vi "CheckZLUTDimensions.vi"(10 "ZLUT":sgl[][][](array[numeric]), 11 "MeasureConfig":T1={"Bead locations"=[{"X"=0, "Y"=0}], "ROI"=200, "Experiment base path"=path "", "Image output subdir"="images", "Output mode"=enum."None", "Traces output subdir"="traces", "QTrk Settings"={"Image width"=150, "Image height"=150, "Number of threads (CPU based)"=-1, "CUDA Device"=-2, "COM Background correction factor"=0.0, "ZLUT MinRadius"=8.0, "ZLUT Radial sample density"=5.0, "ZLUT Angular sample density"=2.0, "ZLUT ROI Coverage"=0.7, "QI Iterations"=1, "QI MinRadius"=2.0, "QI Radial sample density"=5.0, "QI Angular sample density"=2.0, "QI ROI Coverage"=0.7, "QI Angular Step \nIteration Factor"=0.8, "XCOR Profile Length"=1, "XCOR Profile Width"=128, "XCOR Iterations"=32, "Gaussian 2D Fit Iterations"=2, "Gaussian 2D Sigma (pixels)"=3.0, "Downsample"=0}, "Tracking Config"={"Number of steps"=0, "ZLUT stepsize (um)"=0.0, "Z correction factor"=0.0, "Start piezo Z (um)"=0.0, "Pixel size (nm)"=0.0, "2D Localization Type"=enum."Quadrant Interpolation", "Z Command (None)"=enum."Nothing", "Z Piezo scale"=FALSE}, "Experiment Name"="", "Program"={"Commands"=[], "Motor Axis accuracy conditions"={"Magnet Z"=0.0, "Magnet rotation"=0.0, "Camera"={"X"=0.0, "Y"=0.0}, "Piezo XY"={"X"=0.0, "Y"=0.0}, "Piezo Z"=0.0}, "Axis flags"={"Magnet Z"=FALSE, "Magnet rotation"=FALSE, "Camera"={"X"=FALSE, "Y"=FALSE}, "Piezo XY"={"X"=FALSE, "Y"=FALSE}, "Piezo Z"=FALSE}}, "ZLUT"=[], "Camera settings"={"Framerate (Hz)"=60, "Exposure time (us)"=5000, "Image size"={"Width"=1280, "Height"=1024}, "Number of buffers"=30}, "Experiment Script"="", "Max frames in memory"=2, "Save traces as binary"=FALSE, "Pixel Calibration Gain Image"="camera_calib_gain.bin", "Pixel Calibration Offset Image"="camera_calib_gain.bin", "Use pixel calibration images"=FALSE, "Internal camera settings"="", "Trace write interval"=100} {"QTrk Settings"."QI ROI Coverage" format="%_2g"; "QTrk Settings"."QI MinRadius" format="%.2f"; "QTrk Settings"."QI Angular sample density" format="%.3f"; "QTrk Settings"."QI Radial sample density" format="%.2f"; "QTrk Settings"."ZLUT Radial sample density" format="%.2f"; "QTrk Settings"."ZLUT MinRadius" format="%.2f"}) -> (2 "OK?":bool)   [LabVIEW 2011]
uses:
  Typedefs/MeasureConfigType.ctl
  Typedefs/MeasureConfigOutputMode.ctl
  qtrk/QTrkLVBinding/QTrkSettings.ctl
  Typedefs/TrackingConfigType.ctl
  qtrk/QTrkLVBinding/QTrkLocalizationType.ctl
  qtrk/QTrkLVBinding/QTrkZCommandType.ctl
  ExperimentProgram/ExperimentProgramType.ctl
  ExperimentProgram/ExProgCommandType.ctl
  ExperimentProgram/ExProgCommandEnumType.ctl
  Motors/MotorAxisEnum.ctl
  Motors/MotorPosType.ctl
  Typedefs/XYf.ctl
  Motors/MotorPosFlagsType.ctl
  Camera/GenericCameraConfigType.ctl
panel:
  # "(used for commands with string parameters)"
  # "-2: Use all devices\n-1: Use best device"
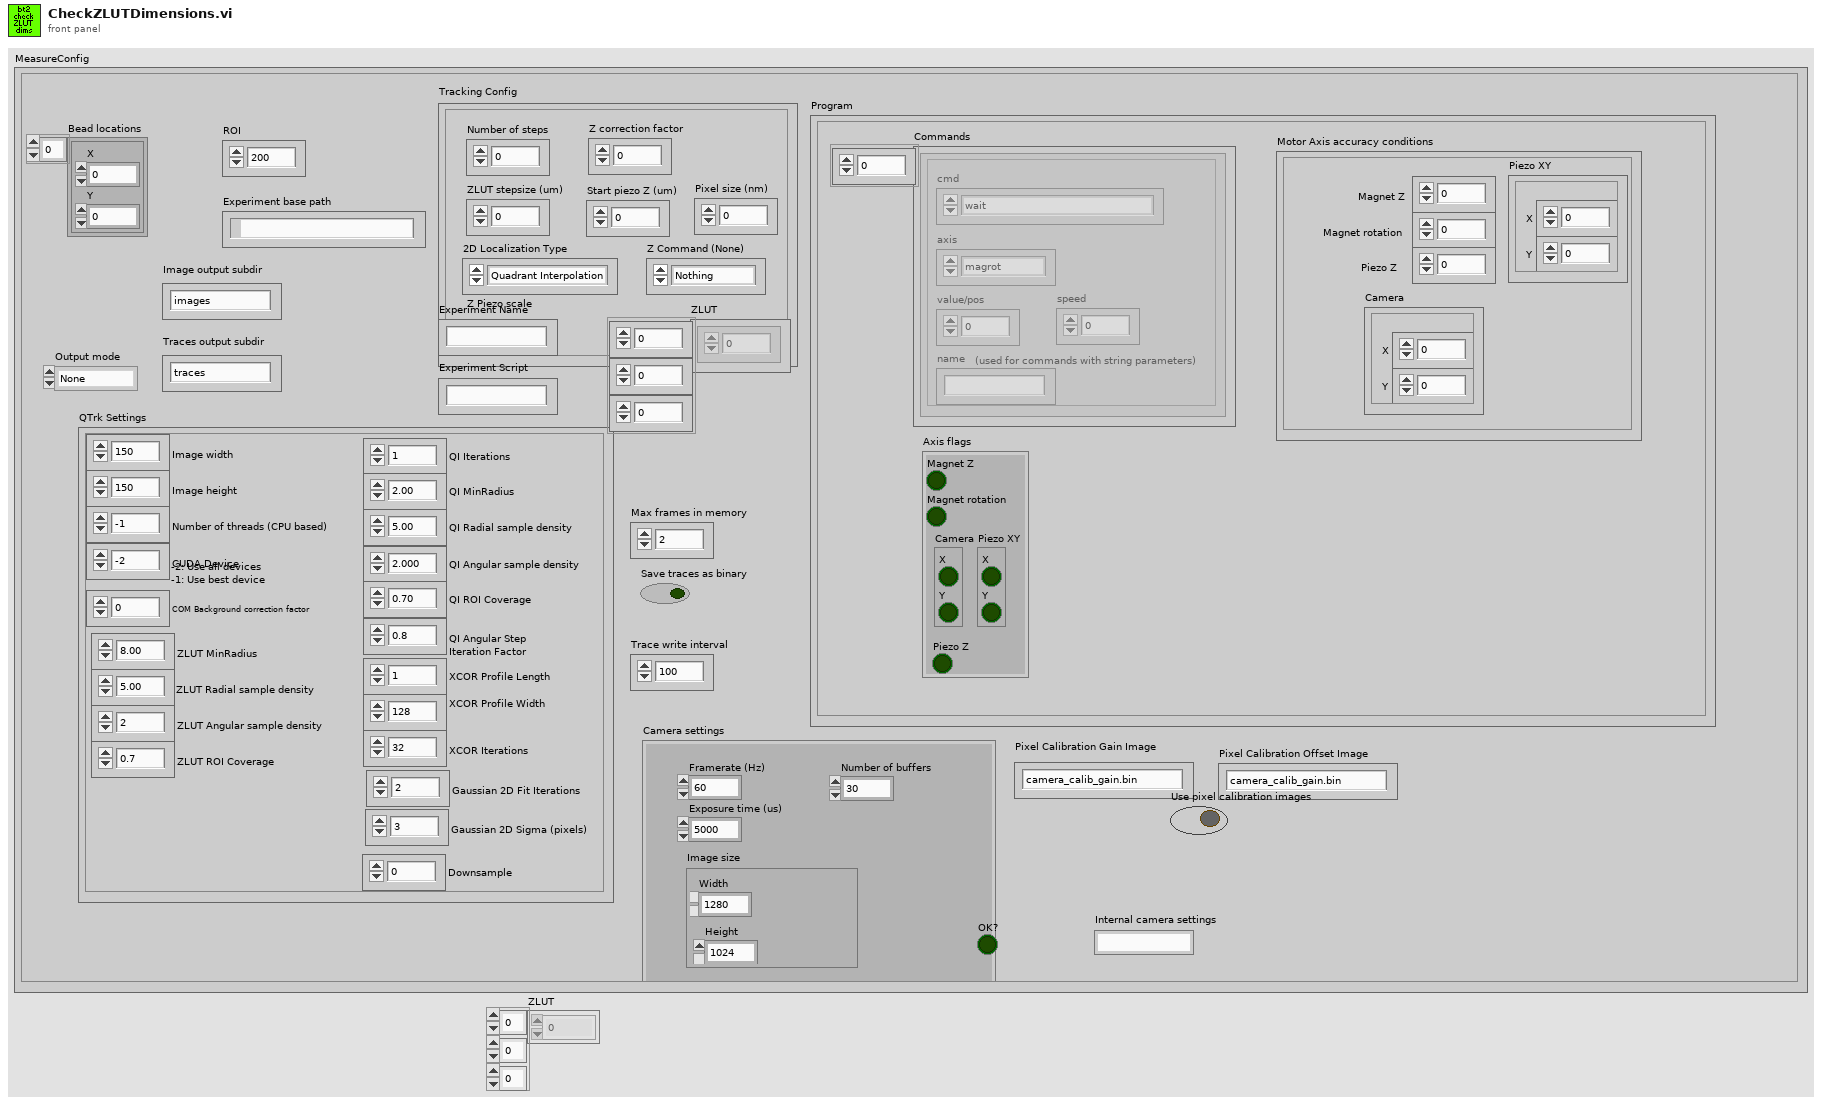
[diagram p1: front panel]
types:
  T1 = typedef "MeasureConfigType.ctl" = cluster{"Bead locations":cluster{"X":i32, "Y":i32}[], "ROI":i32, "Experiment base path":path, "Image output subdir":string, "Output mode":T2, "Traces output subdir":string, "QTrk Settings":T3, "Tracking Config":T4, "Experiment Name":string, "Program":T7, "ZLUT":sgl[][][], "Camera settings":T14, "Experiment Script":string, "Max frames in memory":i32, "Save traces as binary":bool, "Pixel Calibration Gain Image":string, "Pixel Calibration Offset Image":string, "Use pixel calibration images":bool, "Internal camera settings":string, "Trace write interval":i32}
  T2 = typedef "MeasureConfigOutputMode.ctl" = enum16{"None", "Track", "SaveImages"}
  T3 = typedef "QTrkSettings.ctl" = cluster{"Image width":i32, "Image height":i32, "Number of threads (CPU based)":i32, "CUDA Device":i32, "COM Background correction factor":sgl, "ZLUT MinRadius":sgl, "ZLUT Radial sample density":sgl, "ZLUT Angular sample density":sgl, "ZLUT ROI Coverage":sgl, "QI Iterations":i32, "QI MinRadius":sgl, "QI Radial sample density":sgl, "QI Angular sample density":sgl, "QI ROI Coverage":sgl, "QI Angular Step \nIteration Factor":sgl, "XCOR Profile Length":i32, "XCOR Profile Width":i32, "XCOR Iterations":i32, "Gaussian 2D Fit Iterations":i32, "Gaussian 2D Sigma (pixels)":sgl, "Downsample":i32}
  T4 = typedef "TrackingConfigType.ctl" = cluster{"Number of steps":i32, "ZLUT stepsize (um)":sgl, "Z correction factor":sgl, "Start piezo Z (um)":sgl, "Pixel size (nm)":sgl, "2D Localization Type":T5, "Z Command (None)":T6, "Z Piezo scale":bool}
  T5 = typedef "QTrkLocalizationType.ctl" = enum16{"Center-of-Mass", "1D Cross-Correlation", "Quadrant Interpolation", "Gaussian 2D MLE", "QI + ZLUTAlign", "ZLUTAlign", "QI + FourierLUT"}
  T6 = typedef "QTrkZCommandType.ctl" = enum16{"Nothing", "ComputeZ", "BuildRadialZLUT", "BuildImageZLUT", "RadialZLUT+ImageZLUT"}
  T7 = typedef "ExperimentProgramType.ctl" = cluster{"Commands":T8[], "Motor Axis accuracy conditions":T11, "Axis flags":T13}
  T8 = typedef "ExProgCommandType.ctl" = cluster{"cmd":T9, "axis":T10, "value/pos":dbl, "speed":dbl, "name":string}
  T9 = typedef "ExProgCommandEnumType.ctl" = enum16{"wait", "move", "acquire", "idle", "rmove", "when", "section", "stop"}
  T10 = typedef "MotorAxisEnum.ctl" = enum16{"no axis", "magrot", "magpos", "px", "py", "pz", "camx", "camy"}
  T11 = typedef "MotorPosType.ctl" = cluster{"Magnet Z":dbl, "Magnet rotation":dbl, "Camera":T12, "Piezo XY":T12, "Piezo Z":dbl}
  T12 = typedef "XYf.ctl" = cluster{"X":sgl, "Y":sgl}
  T13 = typedef "MotorPosFlagsType.ctl" = cluster{"Magnet Z":bool, "Magnet rotation":bool, "Camera":cluster{"X":bool, "Y":bool}, "Piezo XY":cluster{"X":bool, "Y":bool}, "Piezo Z":bool}
  T14 = typedef "GenericCameraConfigType.ctl" = cluster{"Framerate (Hz)":i32, "Exposure time (us)":i32, "Image size":cluster{"Width":i32, "Height":i32}, "Number of buffers":i32}
  T15 = typedef "QTrkInstance.ctl" = cluster{"QTrk Pointer":u64}
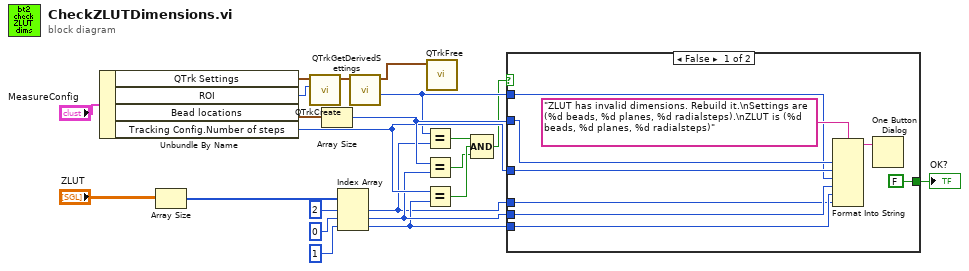
[diagram p0: block diagram]
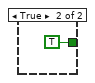
[diagram p2: hidden frame]
diagram:
  n1 = Unbundle By Name("MeasureConfig") -> ("QTrk Settings"=w21:T3, "ROI"=w22:i32, "Bead locations"=w17:cluster{"X":i32, "Y":i32}[], "Tracking Config.Number of steps"=w8:i32)
  n2 = Array Size(array="ZLUT") -> (size(s)=w19:i32[])
  n3 = call "QTrkCreate.vi"("ROI"=w22, "QTrk Settings"=w21) -> ("QTrk Instance"=w11:T15)  [unwired: 3 in, 2 out]
  n4 = Array Size(array=w17) -> (size(s)=w9:i32)
  n5 = Index Array(array=w19, index #1=2 ("index"), index #2=0 ("index"), index #3=1 ("index")) -> (element #1=w4:i32, element #2=w6:i32, element #3=w5:i32)
  n6 = call "QTrkGetDerivedSettings.vi"("QTrk Instance"=w11) -> ("ZLUT Radial Steps"=w7:i32, "QTrk Instance (out)"=w3:T15)  [unwired: 5 in, 4 out]
  n7 = Equal?(x=w7, y=w4) -> (x = y?=w14:bool)
  n8 = Equal?(x=w9, y=w6) -> (x = y?=w12:bool)
  n9 = Equal?(x=w8, y=w5) -> (x = y?=w13:bool)
  n10 = call "QTrkFree.vi"("QTrk Instance"=w3) -> ()  [unwired: 6 in, 1 out]
  n11 = Compound Arithmetic op=AND(w14, w13, w12) -> (w1:bool)
  n12 = case shown="False" w1 {
    tunnel: [FALSE TRUE] -> w10
    tunnel: w9 -> [w29 _]
    tunnel: w8 -> [w28 _]
    tunnel: w7 -> [w27 _]
    tunnel: w6 -> [w26 _]
    tunnel: w5 -> [w25 _]
    tunnel: w4 -> [w24 _]
    frame False {
      n13 = Format Into String(format string="ZLUT has invalid dimensions. Rebuild it.\nSettings are (%d beads, %d planes, %d radialsteps).\nZLUT is (%d beads, %d planes, %d radialsteps)" ("message"), w29, w28, w27, w26, w25, w24) -> (resulting string=w23:string)  [unwired: 2 in, 1 out]
      n14 = One Button Dialog(message=w23) -> ()  [unwired: 1 in, 1 out]
    }
    frame True {
    }
  }
  "OK?" <- w10
